vi "gate sts.vi"() -> ()   [LabVIEW 2010]
uses:
  <userlib>/Nanonis Prog Interface V5/Nanonis Prog Interface.lvlib
panel:
  out "Current Gate Voltage (V)":dbl
  out "Ender":bool
  out "Stop Loop":bool
  in  "Stop":bool
  in  "Increment Gate (V)":dbl
  in  "End Gate (V)":dbl
  in  "Start Gate (V)":dbl
  in  "Basename":string
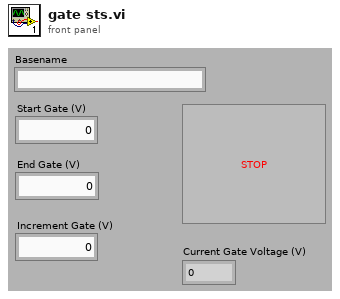
[diagram p1: front panel]
types:
  T1 = cluster{"Save all":enum16{"no change", "on", "off"}, "Number of Sweeps (0=no change)":i32}
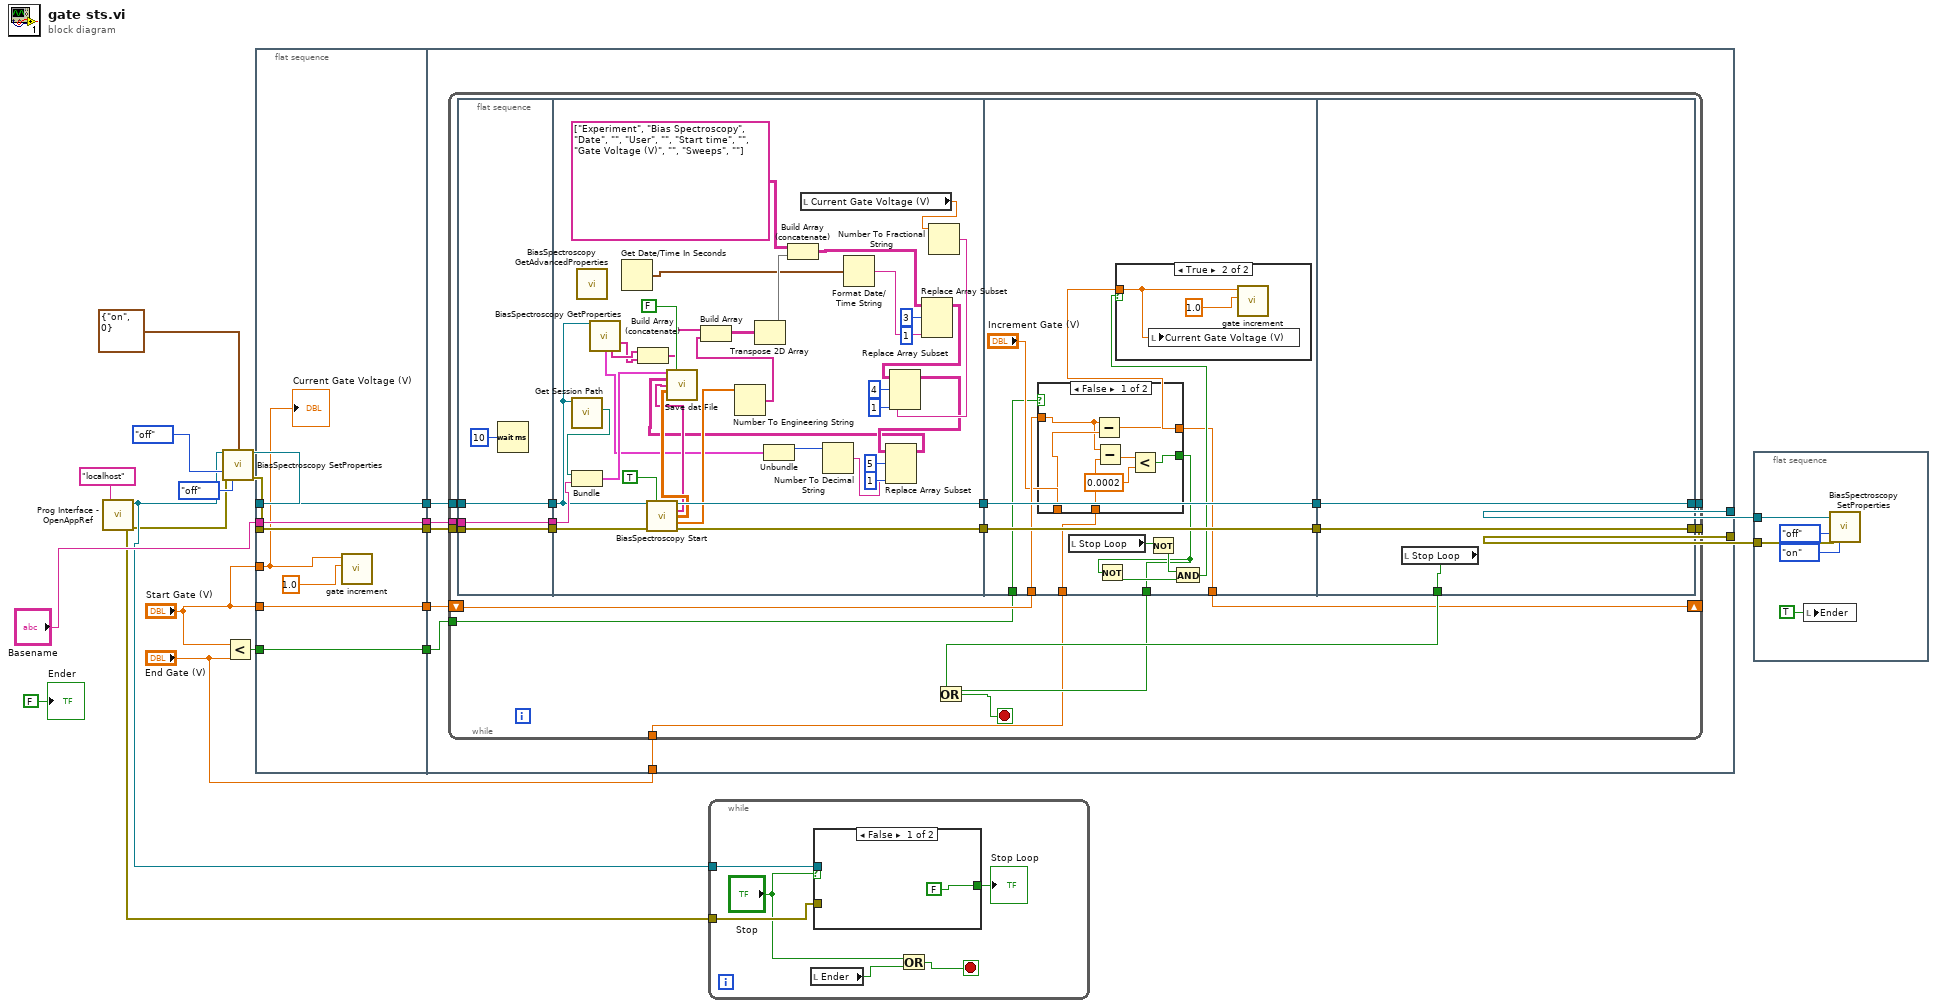
[diagram p0: block diagram]
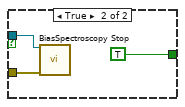
[diagram p2: hidden frame]
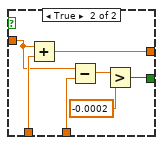
[diagram p3: hidden frame]
diagram:
  n1 = call <userlib>:"Prog Interface - OpenAppRef.vi"("Machine name (local machine IP)"="localhost" ("machine name (localhost)")) -> ("Error out"=w3:errorcluster, "Application reference"=w4:refnum<vi>)  [unwired: 5 in]
  n2 = call <userlib>:"BiasSpectroscopy SetProperties.vi"("Application ref in"=w4, "Autosave (no change)"=enum16{"no change", "on", "off"}."off", "Error in (no error)"=w3, "Save dialog"=enum16{"no change", "on", "off"}."off", "Multiple sweeps config"=T1 {"Save all"=enum."on", "Number of Sweeps (0=no change)"=0}) -> ("Application ref out"=w17:refnum<vi>, "Error out"=w18:errorcluster)  [unwired: 9 in]
  n3 = Less?(x="Start Gate (V)", y="End Gate (V)") -> (x < y?=w12:bool)
  n4 = flat-sequence {
    tunnel: "Start Gate (V)" -> [w23]
    tunnel: w12 -> [w24]
    tunnel: w17 -> [w25]
    tunnel: w18 -> [w26]
    tunnel: "Basename" -> [w27]
    tunnel: [w27] -> w11
    tunnel: [w26] -> w10
    tunnel: [w25] -> w9
    tunnel: [w24] -> w8
    tunnel: [w23] -> w7
    tunnel: "Start Gate (V)" -> [w21]
    tunnel: [w32] -> w15
    tunnel: [w31] -> w14
    tunnel: w11 -> [w35]
    tunnel: w10 -> [w34]
    tunnel: w9 -> [w33]
    tunnel: w8 -> [w30]
    tunnel: w7 -> [w29]
    tunnel: "End Gate (V)" -> [w28]
    frame #0 {
      n5 = call "gate increment.vi"("Increment"=1.0, "Gate Voltage"=w21) -> ()  [unwired: 8 in, 2 out]
      "Current Gate Voltage (V)" <- w21
    }
    frame #1 {
      n6 = while {
        tunnel: w35 -> [w54]
        tunnel: w34 -> [w53]
        tunnel: w33 -> [w52]
        tunnel: [w51] -> w32
        tunnel: [w50] -> w31
        tunnel: w30 -> [w36]
        shift-right: [w40] -> _
        shift-left: w29 -> [w38]
        tunnel: w28 -> [w37]
        stop <- w41 stop-if-true
        n7 = flat-sequence {
          tunnel: w52 -> [w56]
          tunnel: w53 -> [w57]
          tunnel: w54 -> [w58]
          tunnel: [w58] -> w45
          tunnel: [w57] -> w44
          tunnel: [w56] -> w43
          tunnel: [w92] -> w47
          tunnel: [w93] -> w46
          tunnel: w45 -> [w85]
          tunnel: w44 -> [w94]
          tunnel: w43 -> [w84]
          tunnel: [w106] -> w49
          tunnel: [w105] -> w48
          tunnel: w47 -> [w106]
          tunnel: w46 -> [w105]
          tunnel: [w101] -> w40
          tunnel: [w99] -> w39
          tunnel: w38 -> [w98]
          tunnel: w37 -> [w96]
          tunnel: w36 -> [w95]
          tunnel: [w124] -> w51
          tunnel: [w125] -> w50
          tunnel: w49 -> [w125]
          tunnel: w48 -> [w124]
          tunnel: [w123] -> w42
          frame #0 {
            n8 = Wait (ms)(milliseconds to wait=u32 10) -> ()  [unwired: 1 out]
          }
          frame #1 {
            n9 = call <userlib>:"Get Session Path.vi"("Application ref in"=w84) -> ("Session path"=w90:path)  [unwired: 8 in, 2 out]
            n10 = Bundle("Session path"=w90, "Basename"=w85) -> (w89:cluster{"Session path":path, "Basename":string})  [unwired: 1 in]
            n11 = call <userlib>:"BiasSpectroscopy GetAdvancedProperties.vi"() -> ()  [unwired: 10 in, 6 out]
            n12 = call <userlib>:"BiasSpectroscopy GetProperties.vi"("Application ref in"=w84) -> ("Parameters"=w76:string[], "Multiple sweeps configuration"=w65:cluster{"Number of Sweeps":i32, "Save all":bool}, "Fixed parameters"=w77:string[])  [unwired: 7 in, 5 out]
            n13 = Get Date/Time In Seconds() -> (seconds since 1Jan1904=w75:timestamp)
            n14 = Build Array (concatenate)(w77, w76) -> (w81:string[])
            n15 = call <userlib>:"BiasSpectroscopy Start.vi"("Application ref in"=w84, "Get data (F)"=TRUE, "Error in (no error)"=w94) -> ("Application ref out"=w93:refnum<vi>, "Channels"=w87:string[], "Data"=w88:sgl[][], "Parameters"=w83:sgl[], "Error out"=w92:errorcluster)  [unwired: 8 in]
            n16 = Number To Engineering String(4:w83) -> (0:w82:string[])  [unwired: 3 in]
            n17 = Build Array(w81, w82) -> (w80:string[][])
            n18 = Transpose 2D Array(2D array=w80) -> (transposed array=w78:string[][])
            n19 = Unbundle(w65) -> ("Number of Sweeps"=w64:i32)  [unwired: 1 out]
            n20 = Build Array (concatenate)(string[][] [["Experiment", "Bias Spectroscopy"], ["Date", ""], ["User", ""], ["Start time", ""], ["Gate Voltage (V)", ""], ["Sweeps", ""]] ("Attributes"), w78) -> (w74:string[][])
            n21 = local read "Current Gate Voltage (V)"() -> (w67:dbl)
            n22 = Number To Decimal String(number=w64) -> (decimal integer string=w59:string)  [unwired: 1 in]
            n23 = Format Date/Time String(seconds (now)=w75) -> (date/time string=w73:string)  [unwired: 2 in]
            n24 = Replace Array Subset(array=w74, new element=w73, index (row)=3, index (col)=1 ("disabled index (col)")) -> (w70:string[][])
            n25 = Number To Fractional String(number=w67) -> (F-format string=w66:string)  [unwired: 3 in]
            n26 = Replace Array Subset(array=w70, new element=w66, index (row)=4, index (col)=1 ("disabled index (col)")) -> (w63:string[][])
            n27 = Replace Array Subset(array=w63, new element=w59, index (row)=5, index (col)=1 ("disabled index (col)")) -> (w62:string[][])
            n28 = call <userlib>:"Save dat File.vi"("Filename control"=w89, "Show save dialog (T)"=FALSE, "Attributes"=w62, "Channels names"=w87, "Data"=w88) -> ()  [unwired: 7 in, 4 out]
          }
          frame #2 {
            n29 = case shown="False" w95 {
              tunnel: w98 -> [w111 w117]
              tunnel: "Increment Gate (V)" -> [w112 w120]
              tunnel: [w113 w119] -> w101
              tunnel: w96 -> [w110 w118]
              tunnel: [w108 w116] -> w99
              frame False {
                n30 = Subtract(x=w111, y=w112) -> (x-y=w113:dbl)
                n31 = Subtract(x=w111, y=w110) -> (x-y=w109:dbl)
                n32 = Less?(x=w109, y=0.0002) -> (x < y?=w108:bool)
              }
              frame True {
                n33 = Add(x=w117, y=w120) -> (x+y=w119:dbl)
                n34 = Subtract(x=w117, y=w118) -> (x-y=w115:dbl)
                n35 = Greater?(x=w115, y=-0.0002) -> (0:w116:bool)
              }
            }
            n36 = local read "Stop Loop"() -> (w104:bool)
            n37 = Not(x=w99) -> (.not. x?=w100:bool)
            n38 = Not(x=w104) -> (.not. x?=w102:bool)
            n39 = And(x=w102, y=w100) -> (x .and. y?=w103:bool)
            n40 = case shown="True" w103 {
              tunnel: w101 -> [_ w122]
              frame False {
              }
              frame True {
                n41 = local write "Current Gate Voltage (V)"(w122) -> ()
                n42 = call "gate increment.vi"("Increment"=1.0, "Gate Voltage"=w122) -> ()  [unwired: 8 in, 2 out]
              }
            }
          }
          frame #3 {
            n43 = local read "Stop Loop"() -> (w123:bool)
          }
        }
        n44 = Or(x=w39, y=w42) -> (x .or. y?=w41:bool)
      }
    }
  }
  n45 = while {
    tunnel: w4 -> [w131]
    tunnel: w3 -> [w130]
    stop <- w127 stop-if-true
    n46 = local read "Ender"() -> (w126:bool)
    n47 = case shown="False" "Stop" {
      tunnel: w131 -> [_ w135]
      tunnel: w130 -> [_ w134]
      tunnel: [FALSE TRUE] -> w129
      frame False {
      }
      frame True {
        n48 = call <userlib>:"BiasSpectroscopy Stop.vi"("Application ref in"=w135, "Error in (no error)"=w134) -> ()  [unwired: 12 in, 2 out]
      }
    }
    "Stop Loop" <- w129
    n49 = Or(x="Stop", y=w126) -> (x .or. y?=w127:bool)
  }
  n50 = flat-sequence {
    tunnel: w15 -> [w140]
    tunnel: w14 -> [w139]
    frame #0 {
      n51 = local write "Ender"(TRUE ("Ender")) -> ()
      n52 = call <userlib>:"BiasSpectroscopy SetProperties.vi"("Application ref in"=w140, "Autosave (no change)"=enum16{"no change", "on", "off"}."off", "Error in (no error)"=w139, "Save dialog"=enum16{"no change", "on", "off"}."on") -> ()  [unwired: 10 in, 2 out]
    }
  }
  "Ender" <- FALSE ("Ender")
